vi "Get Chamber Status-setup.vi"(11 "test case ID":string) -> (3 "Test Error":errorcluster)   [LabVIEW 2018]
doc: "The setup VI should be executed before the VI under test in the harness VI. In this VI you can prepare the environment and the inputs of the VI under test.\n\nSee the Help Document for more information. (<b>Help</b> > <b>IncQuery Labs</b> > <b>InstaCoverage</b> > <b>InstaCoverage Help...</b>)"
uses:
  Libraries/Thermal Chamber Response Simulator/Thermal Chamber Response Simulator.lvlib
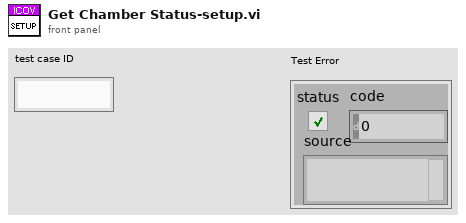
[diagram p1: front panel]
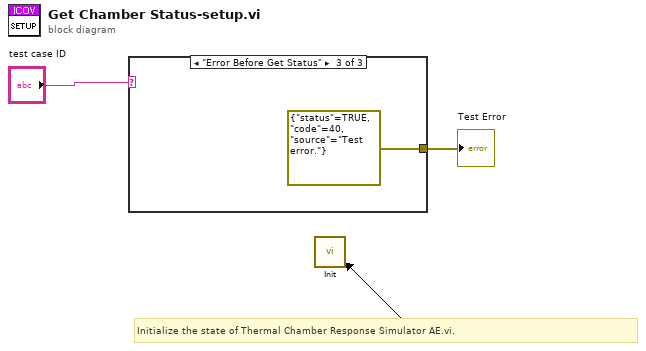
[diagram p0: block diagram]
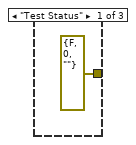
[diagram p2: hidden frame]
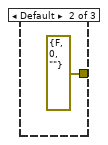
[diagram p3: hidden frame]
diagram:
  # "Initialize the state of Thermal Chamber Response Simulator AE.vi."
  n1 = case shown="\"Error Before Get Status\"" "test case ID" {
    tunnel: [errorcluster {"status"=FALSE, "code"=0, "source"=""} ("Test Error") errorcluster {"status"=FALSE, "code"=0, "source"=""} ("Test Error") errorcluster {"status"=TRUE, "code"=40, "source"="Test error."} ("Test Error")] -> w1
    frame "Test Status" {
    }
    frame Default {
    }
    frame "Error Before Get Status" {
    }
  }
  "Test Error" <- w1
  n2 = call "Init.vi"() -> ()  [unwired: 11 in, 1 out]
